vi "PFI-28000-System_Set Test.vi"(8 "error in (no error)":errorcluster, 10 "Enabled":bool, 11 "PFI-28000-System in":refnum<class "PFI-28000-System.lvclass">) -> (0 "error out":errorcluster, 3 "PFI-28000-System out":refnum<class "PFI-28000-System.lvclass">)   [LabVIEW 2017, in "PFI-28000-System.lvclass"]
uses:
  PFI-28000-System.lvclass
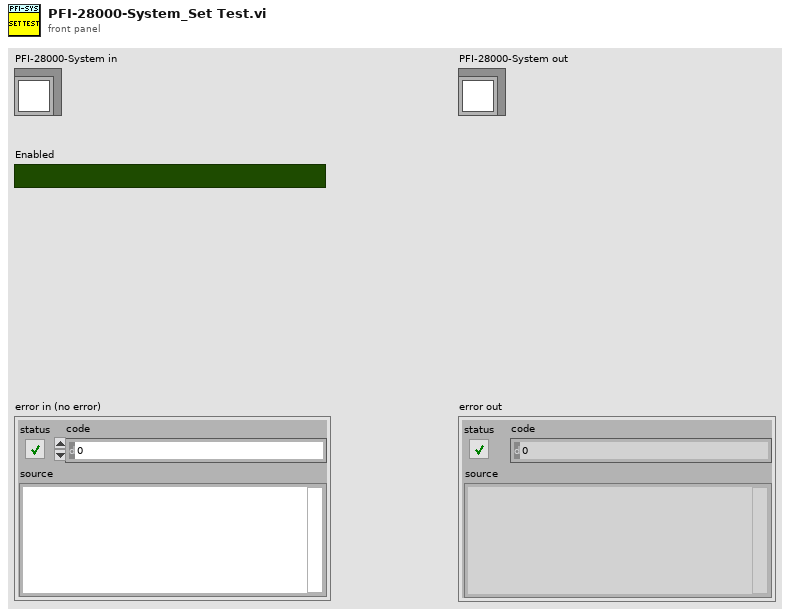
[diagram p1: front panel]
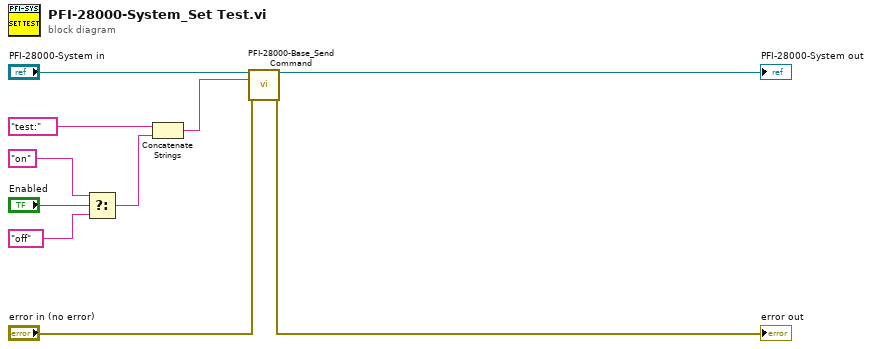
[diagram p0: block diagram]
diagram:
  n1 = Select(t="on" ("Command"), s="Enabled", f="off" ("Command")) -> (s? t:f=w6:string)
  n2 = Concatenate Strings("test:" ("Command"), w6) -> (w3:string)
  n3 = call-dynamic "PFI-28000-Base_Send Command.vi"("PFI-28000-Base in"="PFI-28000-System in", "Command"=w3, "error in (no error)"="error in (no error)") -> ("PFI-28000-Base out"=→"PFI-28000-System out":refnum<class "PFI-28000-System.lvclass">, "error out"=→"error out":errorcluster)  [unwired: 11 in]
